vi "Find Parent of a Directory.vi"(3 "Directory":string) -> (0 "Directory (stripped)":string, 1 "Parent Directory":string)   [LabVIEW 2020, in "AoC 2022.lvlib"]
uses:
  AoC 2022.lvlib
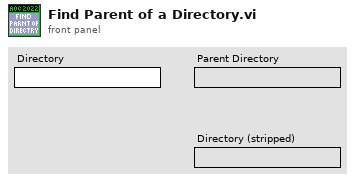
[diagram p1: front panel]
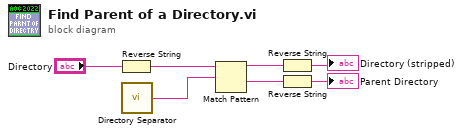
[diagram p0: block diagram]
diagram:
  n1 = Reverse String(1:"Directory") -> (0:w4:string)
  n2 = call "Directory Separator.vi"() -> ("Directory Separator"=w6:string)
  n3 = Match Pattern(string=w4, regular expression=w6) -> (before substring=w2:string, after substring=w3:string)  [unwired: 1 in, 2 out]
  n4 = Reverse String(1:w2) -> (0:→"Directory (stripped)":string)
  n5 = Reverse String(1:w3) -> (0:→"Parent Directory":string)
